vi "Stop Acquisition.vi"(8 "error in (no error)":errorcluster, 11 "HAMAMATSU_DCAMAPI in":refnum<class "HAMAMATSU_DCAMAPI.lvclass">) -> (0 "error out":errorcluster, 3 "HAMAMATSU_DCAMAPI out":refnum<class "HAMAMATSU_DCAMAPI.lvclass">)   [LabVIEW 2020, in "HAMAMATSU_DCAMAPI.lvclass"]
uses:
  HAMAMATSU_DCAMAPI.lvclass
  HAMAMATSU_DCAMAPI.lvclass/HAMAMATSU_DCAMAPI.ctl
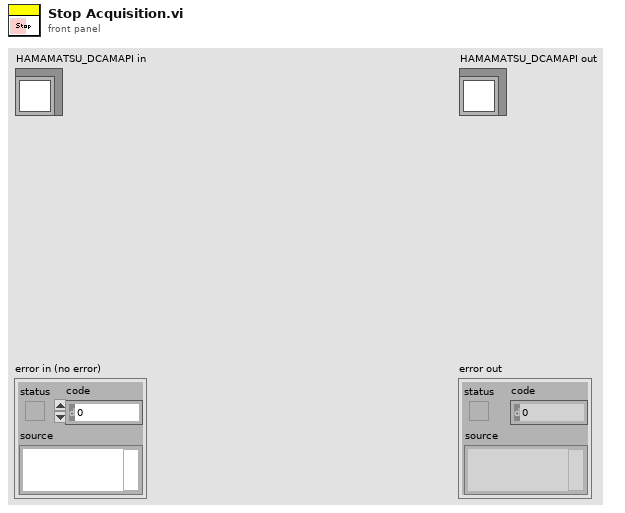
[diagram p1: front panel]
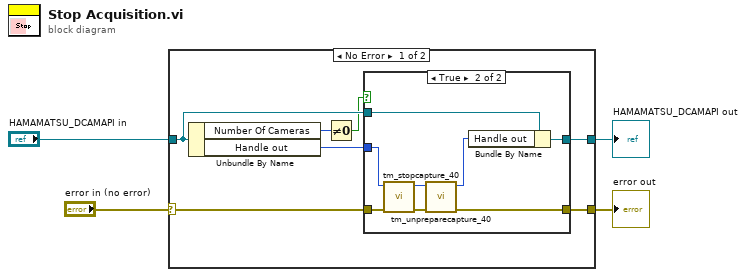
[diagram p0: block diagram]
diagram:
  n1 = case shown="No Error" "error in (no error)" {
    selector: "error in (no error)" -> [w10 w22]
    tunnel: "HAMAMATSU_DCAMAPI in" -> [w8 w23]
    tunnel: [w11 w23] -> w2
    tunnel: [w9 w22] -> w1
    frame No Error {
      n2 = Unbundle By Name(w8) -> ("Number Of Cameras"=w6:u32, "Handle out"=w7:u32)
      n3 = Not Equal To 0?(x=w6) -> (x != 0?=w5:bool)
      n4 = case shown="True" w5 {
        tunnel: w8 -> [w13 w21]
        tunnel: [w13 w15] -> w11
        tunnel: w10 -> [w12 w18]
        tunnel: [w12 w17] -> w9
        tunnel: w7 -> [_ w16]
        frame False {
        }
        frame True {
          n5 = call <userlib>:"tm_stopcapture_40.vi"("error in (no error)"=w18, "Handle in"=w16) -> ("error out"=w19:errorcluster, "Handle out"=w20:u32)  [unwired: 8 in]
          n6 = call <userlib>:"tm_unpreparecapture_40.vi"("error in (no error)"=w19, "Handle in"=w20) -> ("error out"=w17:errorcluster, "Handle out"=w14:u32)  [unwired: 8 in]
          n7 = Bundle By Name(cluster=w21, "Handle out"=w14) -> (w15:refnum<class "HAMAMATSU_DCAMAPI.lvclass">)
        }
      }
    }
    frame Error {
    }
  }
  "error out" <- w1
  "HAMAMATSU_DCAMAPI out" <- w2
